vi "niDTS BT Tx Test INC Default Limits.vi"() -> ()   [LabVIEW 2015, in "niDTS BT.lvlib"]
uses:
  niDTS BT.lvlib
  niDTS BT Tx Test INC IBE Results.ctl
  niDTS BT Tx Test INC Character Results.ctl
  niDTS BT Tx Test INC CFO Resutls.ctl
  niDTS BT Tx Test INC TXP Results.ctl
  niDTS BT Tx Test INC OBW Results.ctl
  niDTS BT Tx Test INC DEVM Results.ctl
  niDTS BT Tx Test INC CF Stability Results.ctl
panel:
  in  "Default USL IBE LE-PT":T1={"Measurement Status"=FALSE, "Reference Channel Power (dBm)"=13.0, "Upper Channel Power (dBm)"=-20.0, "Lower Channel Power (dBm)"=-20.0, "Total Channel Powers (dBm)"=[]}
  in  "Default USL TXP LE-PT":T2={"Average Burst Power (dBm)"=23.0, "Peak Burst Power (dBm)"=20.0, "EdrRelativePower (dB)"=inf}
  in  "Default USL DF1/DF2 LE-PT":T3={"Average df1Avg (Hz)"=275000.0, "Max df1Max (Hz)"=inf, "Min df1Max (Hz)"=inf, "Measurement Status df1"=FALSE, "Average  df2Avg/Average df1Avg"=inf, "Average df2Avg (Hz)"=inf, "Max df2Max (Hz)"=inf, "Min df2Max (Hz)"=inf, "Measurement Status df2"=FALSE}
  in  "Default USL CFO LE-PT":T4={"Max ICFT (Hz)"=150000.0, "Max Carrier Drift (Hz)"=50000.0, "Max Carrier Drift/50us (Hz)"=20000.0, "LE MaxPayloadBlockFreqOffset (Hz)"=inf, "LE MaxCarrierDrift/55us (Hz)"=inf}
  in  "Default LSL IBE LE-PT":T1={"Measurement Status"=FALSE, "Reference Channel Power (dBm)"=-inf, "Upper Channel Power (dBm)"=-inf, "Lower Channel Power (dBm)"=-inf, "Total Channel Powers (dBm)"=[]}
  in  "Default LSL TXP LE-PT":T2={"Average Burst Power (dBm)"=-inf, "Peak Burst Power (dBm)"=-inf, "EdrRelativePower (dB)"=-inf}
  in  "Default LSL DF1/DF2 LE-PT":T3={"Average df1Avg (Hz)"=225000.0, "Max df1Max (Hz)"=-inf, "Min df1Max (Hz)"=-inf, "Measurement Status df1"=FALSE, "Average  df2Avg/Average df1Avg"=-inf, "Average df2Avg (Hz)"=-inf, "Max df2Max (Hz)"=185000.0, "Min df2Max (Hz)"=-inf, "Measurement Status df2"=FALSE}
  in  "Default LSL CFO LE-PT":T4={"Max ICFT (Hz)"=-150000.0, "Max Carrier Drift (Hz)"=-50000.0, "Max Carrier Drift/50us (Hz)"=-20000.0, "LE MaxPayloadBlockFreqOffset (Hz)"=-inf, "LE MaxCarrierDrift/55us (Hz)"=-inf}
  in  "Default LSL TXP EDR":T2={"Average Burst Power (dBm)"=-inf, "Peak Burst Power (dBm)"=-inf, "EdrRelativePower (dB)"=-1.0}
  in  "Default LSL CFS EDR":T5={"Average Inital Freq Error (Hz)"=-75000.0, "Max Initial Freq Error (Hz)"=-75000.0, "Average Block Abs Freq Error (Hz)"=-75000.0, "Max Block Abs Freq Error (Hz)"=-75000.0, "Average Block Rel Freq Error (Hz)"=-10000.0, "MaxBlockRel Freq Error (Hz)"=-10000.0}
  in  "Default LSL DEVM EDR":T6
  in  "Default LSL IBE EDR":T1={"Measurement Status"=FALSE, "Reference Channel Power (dBm)"=-inf, "Upper Channel Power (dBm)"=-inf, "Lower Channel Power (dBm)"=-inf, "Total Channel Powers (dBm)"=[]}
  in  "Default USL TXP EDR":T2={"Average Burst Power (dBm)"=23.0, "Peak Burst Power (dBm)"=20.0, "EdrRelativePower (dB)"=4.0}
  in  "Default USL CFS EDR":T5={"Average Inital Freq Error (Hz)"=75000.0, "Max Initial Freq Error (Hz)"=75000.0, "Average Block Abs Freq Error (Hz)"=75000.0, "Max Block Abs Freq Error (Hz)"=75000.0, "Average Block Rel Freq Error (Hz)"=10000.0, "MaxBlockRel Freq Error (Hz)"=10000.0}
  in  "Default USL DEVM EDR":T6={"Average RMS DEVM (%)"=20.0, "Max Peak DEVM (%)"=35.0, "99% DEVM (%)"=30.0}
  in  "Default USL IBE EDR":T1={"Measurement Status"=FALSE, "Reference Channel Power (dBm)"=23.0, "Upper Channel Power (dBm)"=-20.0, "Lower Channel Power (dBm)"=-20.0, "Total Channel Powers (dBm)"=[]}
  in  "Default USL OBW BDR":T7={"OBW (Hz)"=1500000.0, "Start Frequency (Hz)"=0.0, "Stop Frequency (Hz)"=750000.0} {"Stop Frequency (Hz)" format="%#_8p"; "Start Frequency (Hz)" format="%#_7p"}
  in  "Default USL TXP BDR":T2={"Average Burst Power (dBm)"=20.0, "Peak Burst Power (dBm)"=23.0, "EdrRelativePower (dB)"=inf}
  in  "Default USL CFO BDR":T4={"Max ICFT (Hz)"=75000.0, "Max Carrier Drift (Hz)"=40000.0, "Max Carrier Drift/50us (Hz)"=20000.0, "LE MaxPayloadBlockFreqOffset (Hz)"=nan, "LE MaxCarrierDrift/55us (Hz)"=nan}
  in  "Default USL DF1/DF2 BDR":T3={"Average df1Avg (Hz)"=175000.0, "Max df1Max (Hz)"=inf, "Min df1Max (Hz)"=inf, "Measurement Status df1"=FALSE, "Average  df2Avg/Average df1Avg"=inf, "Average df2Avg (Hz)"=175000.0, "Max df2Max (Hz)"=inf, "Min df2Max (Hz)"=inf, "Measurement Status df2"=FALSE}
  in  "Default USL ACP BDR":T1={"Measurement Status"=FALSE, "Reference Channel Power (dBm)"=23.0, "Upper Channel Power (dBm)"=-20.0, "Lower Channel Power (dBm)"=-20.0, "Total Channel Powers (dBm)"=[]}
  in  "Default LSL OBW BDR":T7={"OBW (Hz)"=0.0, "Start Frequency (Hz)"=-750000.0, "Stop Frequency (Hz)"=0.0} {"Stop Frequency (Hz)" format="%#_4p"; "Start Frequency (Hz)" format="%#_4p"}
  in  "Default LSL TXP BDR":T2={"Average Burst Power (dBm)"=-inf, "Peak Burst Power (dBm)"=-inf, "EdrRelativePower (dB)"=-inf}
  in  "Default LSL CFO BDR":T4={"Max ICFT (Hz)"=-75000.0, "Max Carrier Drift (Hz)"=-40000.0, "Max Carrier Drift/50us (Hz)"=-20000.0, "LE MaxPayloadBlockFreqOffset (Hz)"=nan, "LE MaxCarrierDrift/55us (Hz)"=nan}
  in  "Default LSL DF1/DF2 BDR":T3={"Average df1Avg (Hz)"=140000.0, "Max df1Max (Hz)"=-inf, "Min df1Max (Hz)"=-inf, "Measurement Status df1"=FALSE, "Average  df2Avg/Average df1Avg"=-inf, "Average df2Avg (Hz)"=-inf, "Max df2Max (Hz)"=115000.0, "Min df2Max (Hz)"=0.0, "Measurement Status df2"=FALSE}
  in  "Default LSL ACP BDR":T1={"Measurement Status"=FALSE, "Reference Channel Power (dBm)"=-inf, "Upper Channel Power (dBm)"=-inf, "Lower Channel Power (dBm)"=-inf, "Total Channel Powers (dBm)"=[]}
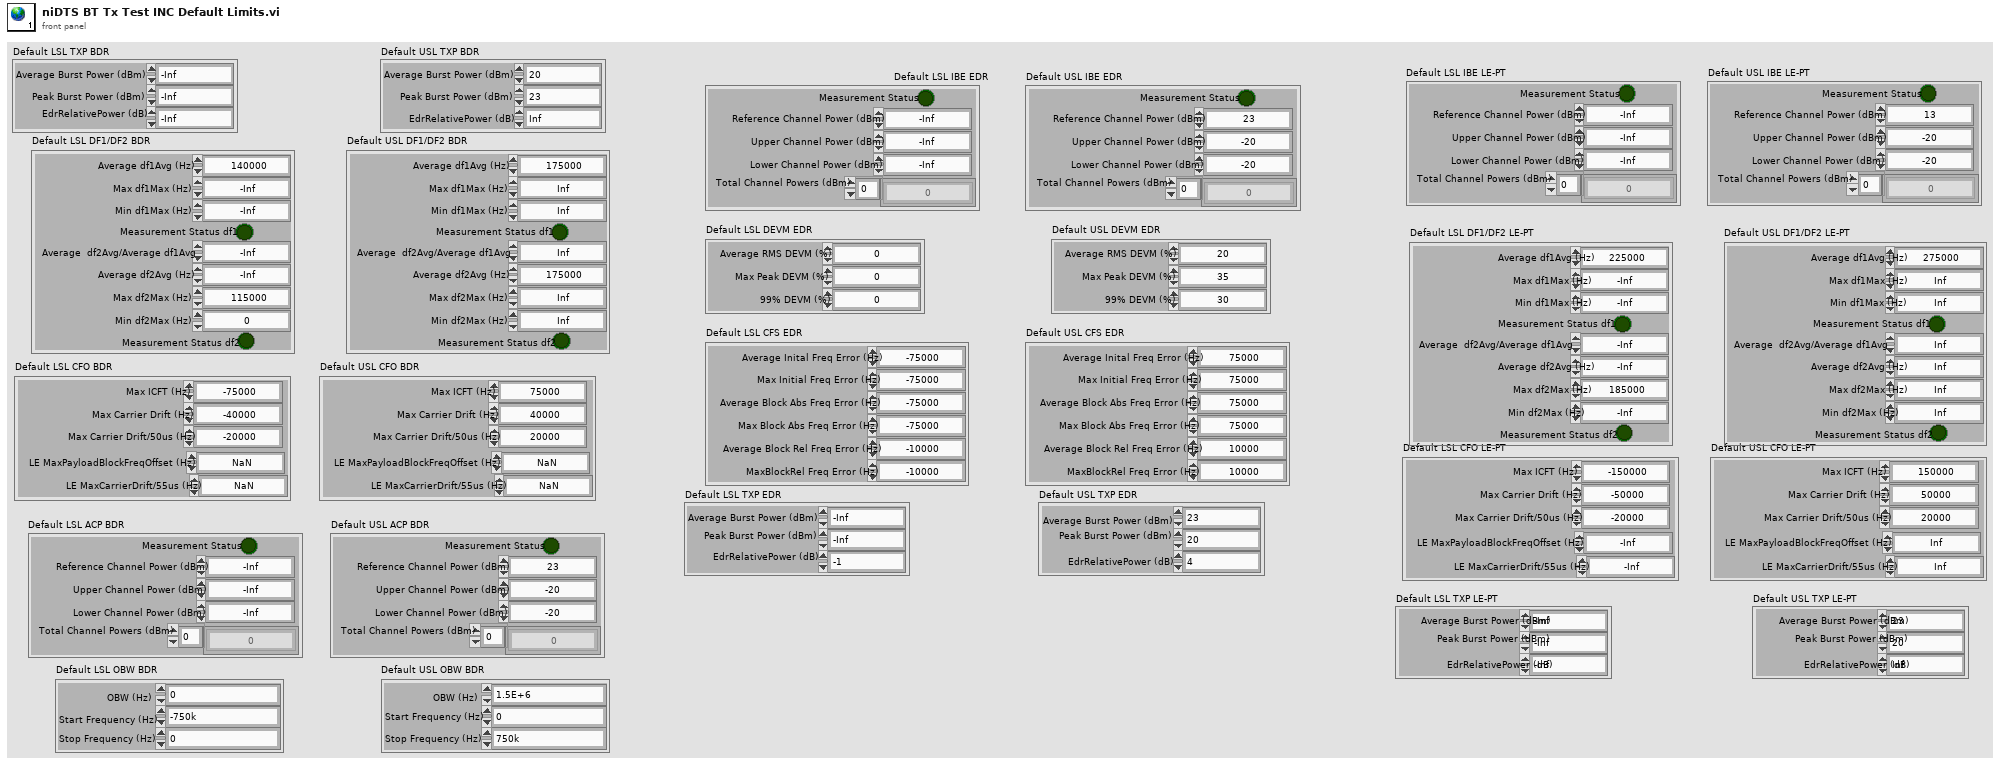
[diagram p1: front panel]
types:
  T1 = typedef "niDTS BT.lvlib/niDTS BT Tx Test INC IBE Results.ctl" = cluster{"Measurement Status":bool, "Reference Channel Power (dBm)":dbl, "Upper Channel Power (dBm)":dbl, "Lower Channel Power (dBm)":dbl, "Total Channel Powers (dBm)":dbl[]}
  T2 = typedef "niDTS BT.lvlib/niDTS BT Tx Test INC TXP Results.ctl" = cluster{"Average Burst Power (dBm)":dbl, "Peak Burst Power (dBm)":dbl, "EdrRelativePower (dB)":dbl}
  T3 = typedef "niDTS BT.lvlib/niDTS BT Tx Test INC Character Results.ctl" = cluster{"Average df1Avg (Hz)":dbl, "Max df1Max (Hz)":dbl, "Min df1Max (Hz)":dbl, "Measurement Status df1":bool, "Average  df2Avg/Average df1Avg":dbl, "Average df2Avg (Hz)":dbl, "Max df2Max (Hz)":dbl, "Min df2Max (Hz)":dbl, "Measurement Status df2":bool}
  T4 = typedef "niDTS BT.lvlib/niDTS BT Tx Test INC CFO Resutls.ctl" = cluster{"Max ICFT (Hz)":dbl, "Max Carrier Drift (Hz)":dbl, "Max Carrier Drift/50us (Hz)":dbl, "LE MaxPayloadBlockFreqOffset (Hz)":dbl, "LE MaxCarrierDrift/55us (Hz)":dbl}
  T5 = typedef "niDTS BT.lvlib/niDTS BT Tx Test INC CF Stability Results.ctl" = cluster{"Average Inital Freq Error (Hz)":dbl, "Max Initial Freq Error (Hz)":dbl, "Average Block Abs Freq Error (Hz)":dbl, "Max Block Abs Freq Error (Hz)":dbl, "Average Block Rel Freq Error (Hz)":dbl, "MaxBlockRel Freq Error (Hz)":dbl}
  T6 = typedef "niDTS BT.lvlib/niDTS BT Tx Test INC DEVM Results.ctl" = cluster{"Average RMS DEVM (%)":dbl, "Max Peak DEVM (%)":dbl, "99% DEVM (%)":dbl}
  T7 = typedef "niDTS BT.lvlib/niDTS BT Tx Test INC OBW Results.ctl" = cluster{"OBW (Hz)":dbl, "Start Frequency (Hz)":dbl, "Stop Frequency (Hz)":dbl}
diagram:
